vi "GetShowInstrNm.vi"(8 "error in (no error)":errorcluster, 11 "BaseDevice in":refnum<class "BaseDevice.lvclass">) -> (0 "error out":errorcluster, 2 "ShowInstrNm":bool[](array[boolean]), 3 "BaseDevice out":refnum<class "BaseDevice.lvclass">)   [LabVIEW 2019, in "BaseDevice.lvclass"]
uses:
  BaseDevice.lvclass
  BaseDevice.lvclass/BaseDevice.ctl
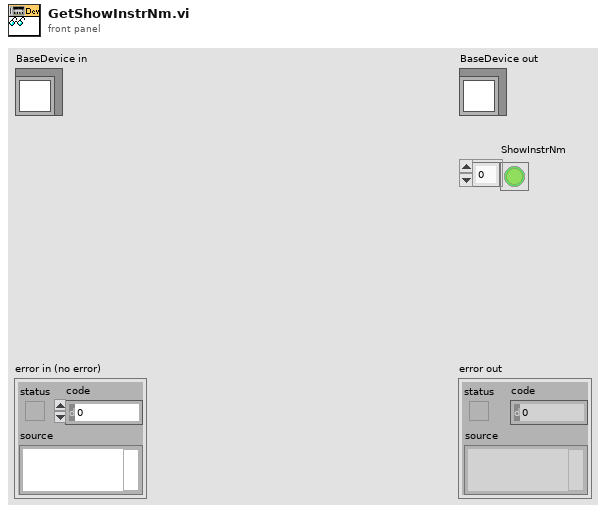
[diagram p1: front panel]
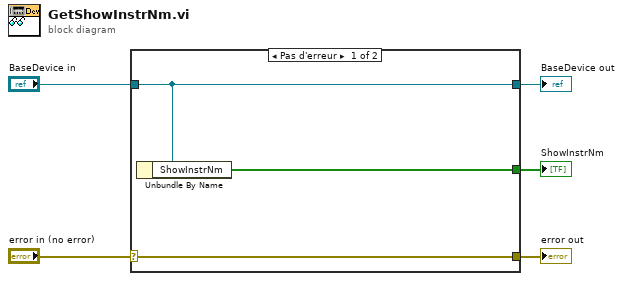
[diagram p0: block diagram]
diagram:
  n1 = case shown="Pas d'erreur" "error in (no error)" {
    selector: "error in (no error)" -> [w8 w9]
    tunnel: [w8 w9] -> w4
    tunnel: [w7 w10] -> w2
    tunnel: "BaseDevice in" -> [w7 w10]
    tunnel: [w6 _] -> w1
    frame No Error {
      n2 = Unbundle By Name(w7) -> ("ShowInstrNm"=w6:bool[])
    }
    frame Error {
    }
  }
  "error out" <- w4
  "BaseDevice out" <- w2
  "ShowInstrNm" <- w1
